vi "Blink3cycle.vi"() -> ()   [LabVIEW 2015]
uses:
  <vilib>/DAQmx/write.llb/DAQmx Write (Analog DBL 1Chan 1Samp).vi
  <vilib>/DAQmx/miscellaneous.llb/DAQmx Fill In Error Info.vi
panel:
  out "error of A1":errorcluster
  out "error of A0":errorcluster
  in  "IamA0 GREEN":refnum<k21>="IamA1"
  in  "IamA1 RED":refnum<k21>="IamA1"
  in  "Stop Button":bool
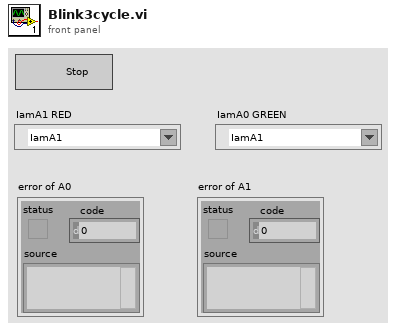
[diagram p1: front panel]
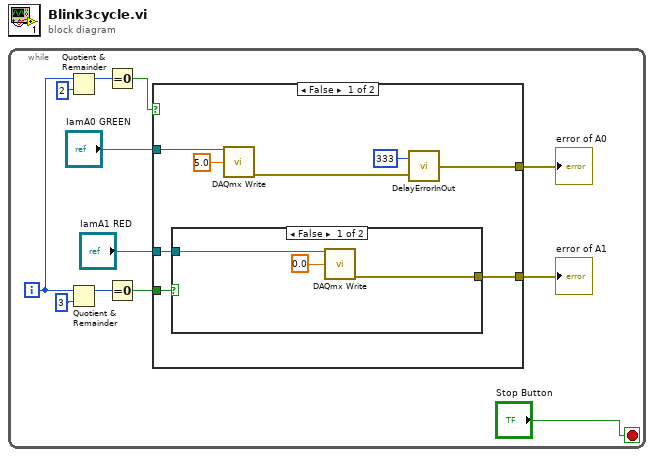
[diagram p0: block diagram]
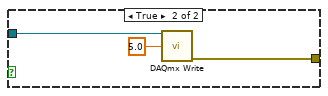
[diagram p2: hidden frame]
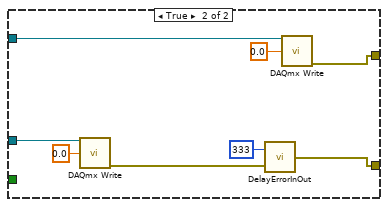
[diagram p3: hidden frame]
diagram:
  n1 = while {
    i -> [w9]
    stop <- "Stop Button" stop-if-true
    n2 = Quotient & Remainder(x=w9, y=2) -> (x-y*floor(x/y)=w10:i32)  [unwired: 1 out]
    n3 = Quotient & Remainder(x=w9, y=3) -> (x-y*floor(x/y)=w7:i32)  [unwired: 1 out]
    n4 = Equal To 0?(x=w10) -> (x = 0?=w6:bool)
    n5 = Equal To 0?(x=w7) -> (x = 0?=w3:bool)
    n6 = case shown="False" w6 {
      tunnel: "IamA0 GREEN" -> [w14 w31]
      tunnel: "IamA1 RED" -> [w15 w30]
      tunnel: [w16 w29] -> w5
      tunnel: [w19 w28] -> w4
      tunnel: w3 -> [w20 _]
      frame False {
        n7 = case shown="False" w20 {
          tunnel: w15 -> [w23 w25]
          tunnel: [w22 w26] -> w19
          frame False {
            n8 = call-poly <vilib>:"DAQmx Write.vi"("task/channels in"=w23, "data"=0.0 ("Voltage (red)")) -> ("error out"=w22:errorcluster)  [unwired: 11 in, 2 out]
          }
          frame True {
            n9 = call-poly <vilib>:"DAQmx Write.vi"("task/channels in"=w25, "data"=5.0 ("Voltage (red)")) -> ("error out"=w26:errorcluster)  [unwired: 11 in, 2 out]
          }
        }
        n10 = call-poly <vilib>:"DAQmx Write.vi"("task/channels in"=w14, "data"=5.0 ("Voltage (red)")) -> ("error out"=w17:errorcluster)  [unwired: 11 in, 2 out]
        n11 = call "DelayErrorInOut.vi"("error in"=w17, "milliseconds to wait"=u32 333) -> ("error out"=w16:errorcluster)
      }
      frame True {
        n12 = call-poly <vilib>:"DAQmx Write.vi"("task/channels in"=w30, "data"=0.0 ("Voltage (red)")) -> ("error out"=w32:errorcluster)  [unwired: 11 in, 2 out]
        n13 = call "DelayErrorInOut.vi"("error in"=w32, "milliseconds to wait"=u32 333) -> ("error out"=w28:errorcluster)
        n14 = call-poly <vilib>:"DAQmx Write.vi"("task/channels in"=w31, "data"=0.0 ("Voltage (red)")) -> ("error out"=w29:errorcluster)  [unwired: 11 in, 2 out]
      }
    }
    "error of A0" <- w5
    "error of A1" <- w4
  }
